vi "PingPong BRAM SM.vi"(6 "Reverse Read?":bool, 8 "Input Valid":bool, 10 "Line Status In":T2, 11 "Input":i16[](array[numeric])=[0, 0, 0, 0]) -> (0 "BRAM Bank0 Write?":bool, 1 "Read Info":cluster{"Read Address":u16, "Read Valid":bool}, 2 "Write Info":cluster{"Write Address":u16, "Write Valid":bool}, 3 "Frame Data Out":T3, 4 "Line Status Out":T2)   [LabVIEW 2014]
uses:
  Acquisition Engine/Acquisition Status.ctl
panel:
  # "Copyright 2014 Vidrio Technologies\nScanImage 5 software is licensed under the Apache License, Version 2.0 (the \"License\"); you may not use any files contained\nwithin the ScanImage 5 release except in compliance with the License. You may obtain a copy of the License at\n http://www.apache.org/licenses/LICENSE-2.0\nUnless required by applicable law or agreed to in writing, software distributed under the License is distributed on an\n\"AS IS\" BASIS, WITHOUT WARRANTIES OR CONDITIONS OF ANY KIND, either express or implied. See the License for the\n specific language governing permissions and limitations under the License."
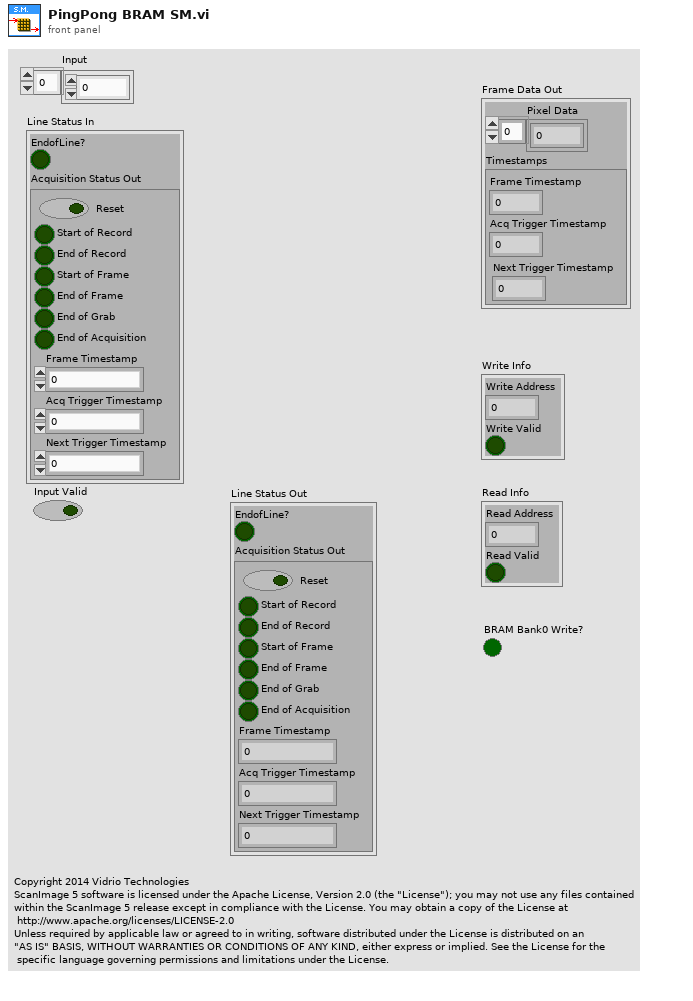
[diagram p1: front panel]
types:
  T1 = typedef "Acquisition Status.ctl" = cluster{"Reset":bool, "Start of Record":bool, "End of Record":bool, "Start of Frame":bool, "End of Frame":bool, "End of Grab":bool, "End of Acquisition":bool, "Frame Timestamp":u64, "Acq Trigger Timestamp":u64, "Next Trigger Timestamp":u64}
  T2 = cluster{"EndofLine?":bool, "Acquisition Status Out":T1}
  T3 = cluster{"Pixel Data":i16[], "Timestamps":cluster{"Frame Timestamp":u64, "Acq Trigger Timestamp":u64, "Next Trigger Timestamp":u64}}
  T4 = cluster{"Frame Timestamp":u64, "Acq Trigger Timestamp":u64, "Next Trigger Timestamp":u64}
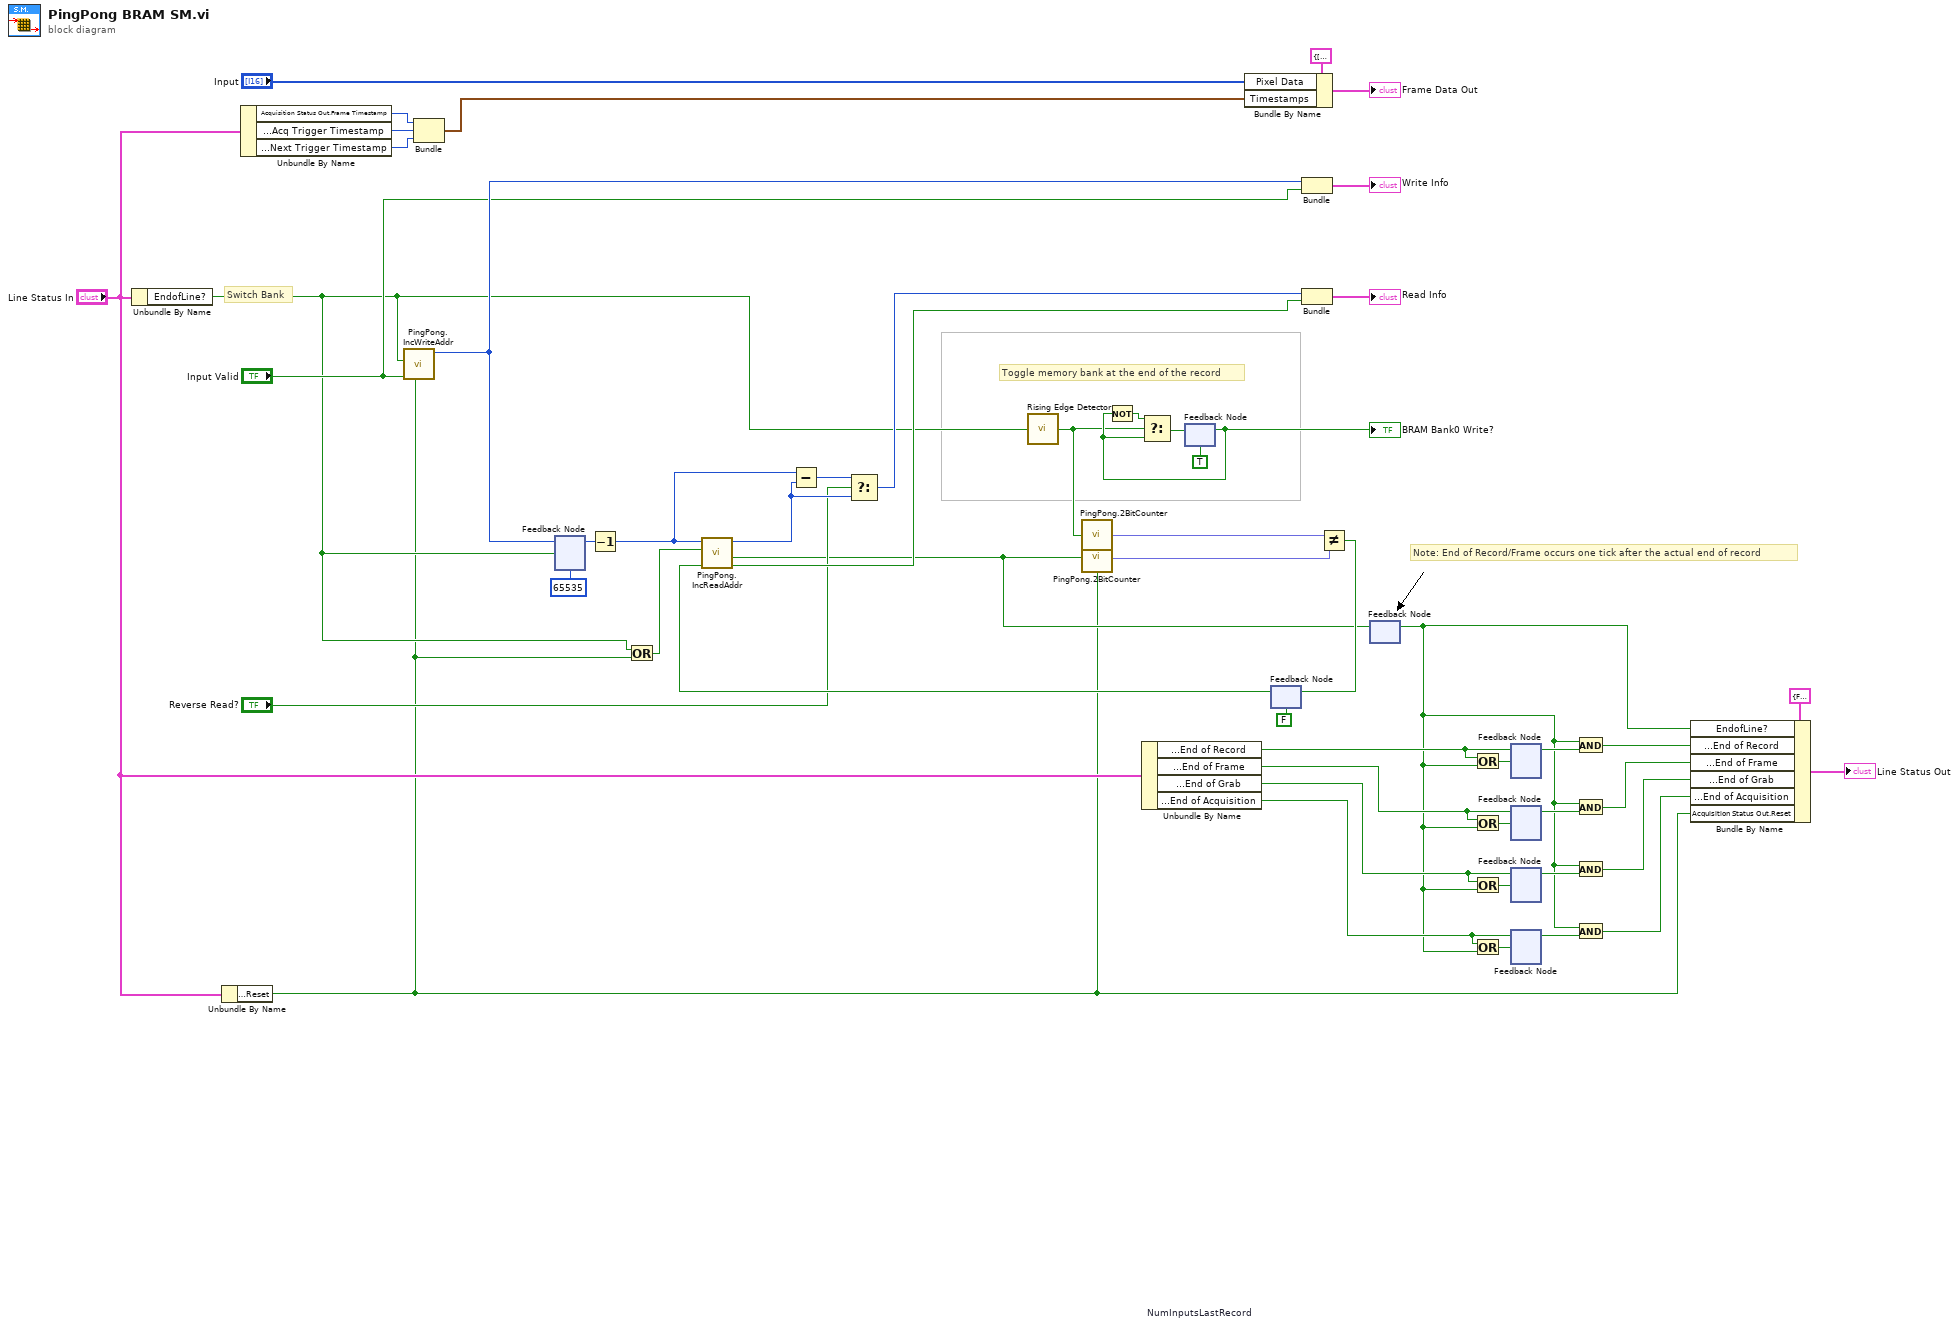
[diagram p0: block diagram]
diagram:
  # "Switch Bank"
  # "Note: End of Record/Frame occurs one tick after the actual end of record"
  # "Toggle memory bank at the end of the record"
  n1 = Unbundle By Name("Line Status In") -> ("EndofLine?"=w27:bool)
  n2 = Unbundle By Name("Line Status In") -> ("Acquisition Status Out.Reset"=w12:bool)
  n3 = Unbundle By Name("Line Status In") -> ("Acquisition Status Out.Frame Timestamp"=w23:u64, "Acquisition Status Out.Acq Trigger Timestamp"=w22:u64, "Acquisition Status Out.Next Trigger Timestamp"=w11:u64)
  n4 = call "PingPong.IncWriteAddr.vi"("Reset"=w12, "INC?"="Input Valid", "End of Line"=w27) -> ("count"=w44:u16)  [unwired: 7 in, 1 out]
  n5 = Bundle("Frame Timestamp"=w23, "Acq Trigger Timestamp"=w22, "Next Trigger Timestamp"=w11) -> (w21:T4)  [unwired: 1 in]
  n6 = feedback-in #1(w44, w27) -> ()
  n7 = feedback #1 "NumInputsLastRecord"(u16 65535 ("count")) -> (w40:u16)
  n8 = Decrement(x=w40) -> (x-1=w34:u16)
  n9 = Or(x=w27, y=w12) -> (x .or. y?=w28:bool)
  n10 = call "Rising Edge Detector.vi"("signal"=w27) -> ("edge detected"=w30:bool)  [unwired: 14 in]
  n11 = call "PingPong.2BitCounter.vi"("Increment"=w30, "Reset"=w12) -> ("Counter Value"=w46:fxp<+,2,2>)  [unwired: 13 in]
  n12 = Unbundle By Name("Line Status In") -> ("Acquisition Status Out.End of Record"=w26:bool, "Acquisition Status Out.End of Frame"=w17:bool, "Acquisition Status Out.End of Grab"=w5:bool, "Acquisition Status Out.End of Acquisition"=w4:bool)
  n13 = feedback #2(TRUE) -> (w53:bool)
  "BRAM Bank0 Write?" <- w53
  n14 = Not(x=w53) -> (.not. x?=w49:bool)
  n15 = Select(t=w49, s=w30, f=w53) -> (s? t:f=w50:bool)
  n16 = feedback-in #2(w50) -> ()
  n17 = Bundle By Name(cluster=T3 {"Pixel Data"=[0, 0, 0, 0], "Timestamps"={"Frame Timestamp"=0, "Acq Trigger Timestamp"=0, "Next Trigger Timestamp"=0}} ("Frame Data Out"), "Pixel Data"="Input", "Timestamps"=w21) -> (→"Frame Data Out":T3)
  n18 = feedback #3(FALSE) -> (w52:bool)
  n19 = call "PingPong.IncReadAddr.vi"("INC?"=w52, "Reset?"=w28, "rollover"=w34) -> ("Output Valid"=w41:bool, "roll over"=w29:bool, "count"=w38:u16)  [unwired: 6 in]
  n20 = Subtract(x=w34, y=w38) -> (x-y=w39:u16)
  n21 = Select(t=w39, s="Reverse Read?", f=w38) -> (s? t:f=w36:u16)
  n22 = call "PingPong.2BitCounter.vi"("Increment"=w29, "Reset"=w12) -> ("Counter Value"=w48:fxp<+,2,2>)  [unwired: 13 in]
  n23 = Bundle("count"=w44, "Input Valid"="Input Valid") -> (→"Write Info":cluster{"count":u16, "Input Valid":bool})  [unwired: 1 in]
  n24 = Bundle("count"=w36, "Output Valid"=w41) -> (→"Read Info":cluster{"count":u16, "Output Valid":bool})  [unwired: 1 in]
  n25 = Not Equal?(x=w46, y=w48) -> (x != y?=w31:bool)
  n26 = feedback-in #3(w31) -> ()
  n27 = feedback #4() -> (w3:bool)  [unwired: 1 in]
  n28 = feedback-in #4(w29) -> ()
  n29 = Or(x=w26, y=w3) -> (x .or. y?=w33:bool)
  n30 = Or(x=w17, y=w3) -> (x .or. y?=w18:bool)
  n31 = Or(x=w5, y=w3) -> (x .or. y?=w9:bool)
  n32 = Or(x=w4, y=w3) -> (x .or. y?=w6:bool)
  n33 = feedback-in #5(w26, w33) -> ()
  n34 = feedback #5() -> (w32:bool)  [unwired: 1 in]
  n35 = feedback #6() -> (w19:bool)  [unwired: 1 in]
  n36 = feedback-in #6(w17, w18) -> ()
  n37 = feedback #7() -> (w8:bool)  [unwired: 1 in]
  n38 = feedback-in #7(w5, w9) -> ()
  n39 = feedback #8() -> (w7:bool)  [unwired: 1 in]
  n40 = feedback-in #8(w4, w6) -> ()
  n41 = And(x=w3, y=w32) -> (x .and. y?=w15:bool)
  n42 = And(x=w3, y=w19) -> (x .and. y?=w14:bool)
  n43 = And(x=w3, y=w8) -> (x .and. y?=w2:bool)
  n44 = And(x=w3, y=w7) -> (x .and. y?=w1:bool)
  n45 = Bundle By Name(cluster=T2 {"EndofLine?"=FALSE, "Acquisition Status Out"={"Reset"=FALSE, "Start of Record"=FALSE, "End of Record"=FALSE, "Start of Frame"=FALSE, "End of Frame"=FALSE, "End of Grab"=FALSE, "End of Acquisition"=FALSE, "Frame Timestamp"=0, "Acq Trigger Timestamp"=0, "Next Trigger Timestamp"=0}} ("Line Status Out 2"), "EndofLine?"=w3, "Acquisition Status Out.End of Record"=w15, "Acquisition Status Out.End of Frame"=w14, "Acquisition Status Out.End of Grab"=w2, "Acquisition Status Out.End of Acquisition"=w1, "Acquisition Status Out.Reset"=w12) -> (→"Line Status Out":T2)
